vi "ElevatedPass.vi"(8 "error in (no error)":errorcluster, 11 "ElevatedPassMode":T1) -> (0 "error out":errorcluster)   [LabVIEW 2013]
doc: "Automatically performs the \"Elevated Pass\" maneuver."
uses:
  ElevatedPassMode.ctl
  DoubleSolenoidAction.ctl
  RollerAction.ctl
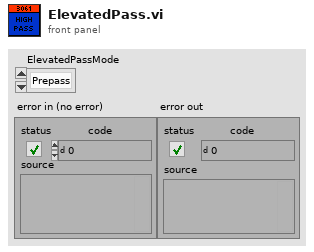
[diagram p1: front panel]
types:
  T1 = typedef "ElevatedPassMode.ctl" = enum16{"Prepass", "Pass", "Stop"}
  T2 = typedef "RollerAction.ctl" = enum16{"Init", "Off", "Forward", "Reverse"}
  T3 = typedef "DoubleSolenoidAction.ctl" = enum16{"Init", "Middle", "In", "Out"}
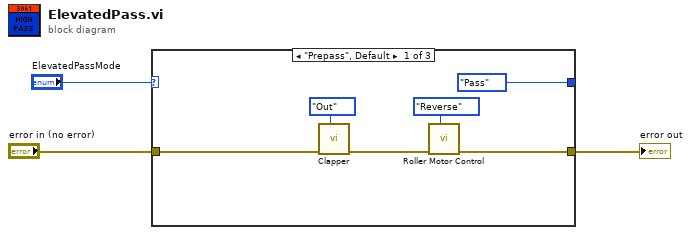
[diagram p0: block diagram]
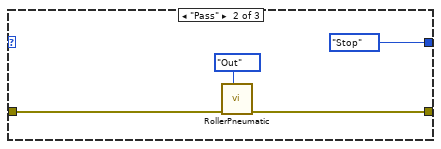
[diagram p2: hidden frame]
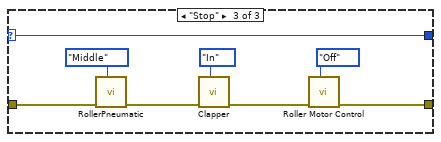
[diagram p3: hidden frame]
diagram:
  n1 = case shown="\"Prepass\", Default" "ElevatedPassMode" {
    selector: "ElevatedPassMode" -> [_ _ w14]
    tunnel: "error in (no error)" -> [w8 w12 w16]
    tunnel: [w5 w11 w15] -> w2
    tunnel: [ElevatedPassMode."Pass" ("ElevatedPassMode") ElevatedPassMode."Stop" ("ElevatedPassMode") w14] -> _
    frame "Prepass", Default {
      n2 = call "Clapper.vi"("State"=DoubleSolenoidAction."Out", "Error in"=w8) -> ("Error out"=w6:errorcluster)  [unwired: 9 in]
      n3 = call "Roller Motor Control.vi"("Action"=RollerAction."Reverse", "Error in"=w6) -> ("Error out"=w5:errorcluster)  [unwired: 9 in]
    }
    frame "Pass" {
      n4 = call "RollerPneumatic.vi"("State"=DoubleSolenoidAction."Out", "Error in"=w12) -> ("Error out"=w11:errorcluster)  [unwired: 9 in]
    }
    frame "Stop" {
      n5 = call "RollerPneumatic.vi"("State"=DoubleSolenoidAction."Middle", "Error in"=w16) -> ("Error out"=w17:errorcluster)  [unwired: 9 in]
      n6 = call "Clapper.vi"("State"=DoubleSolenoidAction."In", "Error in"=w17) -> ("Error out"=w18:errorcluster)  [unwired: 9 in]
      n7 = call "Roller Motor Control.vi"("Action"=RollerAction."Off", "Error in"=w18) -> ("Error out"=w15:errorcluster)  [unwired: 9 in]
    }
  }
  "error out" <- w2
